vi "6.1 Cluster to CSM API String.vi"() -> ()   [LabVIEW 2017]
doc: "### 6.1 Cluster to CSM API String.vi\n\n#### Overview\n\nDemonstrates API String expression for a cluster.\n\n#### Introduction\n\nA cluster is a complex type composed of other data types. This example shows API String expression for clusters. In an API String, a cluster can be expressed in the following two ways:\n\n1. **Tag:Value Mode** In Tag:Value mode, the input string consists of multiple tag-value pairs. A colon (`:`) separates the tag and data, and a semicolon (`;`) separates different elements. Curly braces (`{` and `}`) are used as boundary symbols. For non-complex mixed data types, curly braces can be omitted.\n2. **No-Tag Mode** Clusters also support inputting only data strings, with values separated by semicolons.\n\n#### Steps\n\n- step1: Tag:Value Mode.\n- step2: No-Tag Mode."
uses:
  601d0760-d4b8-4795-a453-687868710894.vi
  39620bd7-9c21-4071-a996-c10094c7c5f6.vi
  6aef6293-1b46-43cc-a090-3bd41170cef4.vi
  c2ea3052-9718-4095-9bf2-a156dcd4a46a.vi
  addons/API-String-Arugments-Support/_Support/Data To API String Arguments.vi
  addons/API-String-Arugments-Support/_Support/Convert API String Arguments to Data(variant).vi
panel:
  out "output cluster":T1={"Data 8"={"Name"="abc", "Child"={"Name"="xxx"}, "Bool"=TRUE}, "Reference cluster in Flatten"={"Name"="abc", "Child"={"Name"="ddd"}, "Bool"=FALSE}, "Flattened String"="{Child.Name:xxx;Bool:TRUE}", "Reference cluster in Retrieve"={"Name"="abc", "Child"={"Name"="ddd"}, "Bool"=FALSE}, "Retrieved Data"={"Name"="abc", "Child"={"Name"="xxx"}, "Bool"=TRUE}}
  out "Flatten Without Reference Cluster":T2={"Original Data"={"Name"="abc", "Child"={"Name"="ddd"}, "Bool"=FALSE}, "Default Reference in Flatten"=variant, "Flattened String"="{Name:abc;Child.Name:ddd;Bool:FALSE}", "Reference cluster in Retrieve"={"Name"="abc", "Child"={"Name"="ddd"}, "Bool"=FALSE}, "Retrieved Data"={"Name"="abc", "Child"={"Name"="ddd"}, "Bool"=FALSE}}
  # "#CSM-Example Overview\n\nDemonstrates API String expression for a cluster."
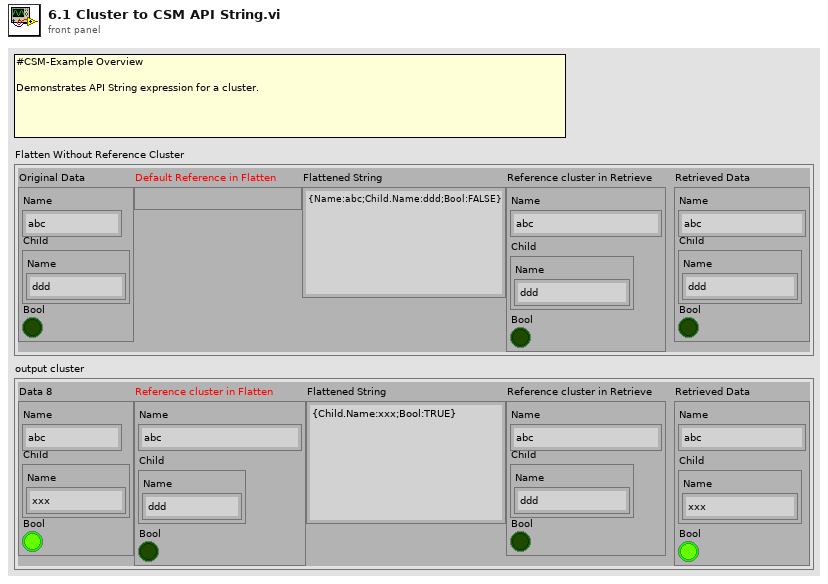
[diagram p1: front panel]
types:
  T1 = cluster{"Data 8":cluster{"Name":string, "Child":cluster{"Name":string}, "Bool":bool}, "Reference cluster in Flatten":cluster{"Name":string, "Child":cluster{"Name":string}, "Bool":bool}, "Flattened String":string, "Reference cluster in Retrieve":cluster{"Name":string, "Child":cluster{"Name":string}, "Bool":bool}, "Retrieved Data":cluster{"Name":string, "Child":cluster{"Name":string}, "Bool":bool}}
  T2 = cluster{"Original Data":cluster{"Name":string, "Child":cluster{"Name":string}, "Bool":bool}, "Default Reference in Flatten":variant, "Flattened String":string, "Reference cluster in Retrieve":cluster{"Name":string, "Child":cluster{"Name":string}, "Bool":bool}, "Retrieved Data":cluster{"Name":string, "Child":cluster{"Name":string}, "Bool":bool}}
  T3 = cluster{"Name":string, "Child":cluster{"Name":string}, "Bool":bool}
  T4 = cluster{"Data 8":cluster{"Name":string, "Child":cluster{"Name":string}, "Bool":bool}, "reference cluster data":variant, "API String":string, "Reference cluster data":cluster{"Name":string, "Child":cluster{"Name":string}, "Bool":bool}, "Data":cluster{"Name":string, "Child":cluster{"Name":string}, "Bool":bool}}
  T5 = cluster{"Data 8":cluster{"Name":string, "Child":cluster{"Name":string}, "Bool":bool}, "Reference cluster data":cluster{"Name":string, "Child":cluster{"Name":string}, "Bool":bool}, "API String":string, "Reference cluster data":cluster{"Name":string, "Child":cluster{"Name":string}, "Bool":bool}, "Data":cluster{"Name":string, "Child":cluster{"Name":string}, "Bool":bool}}
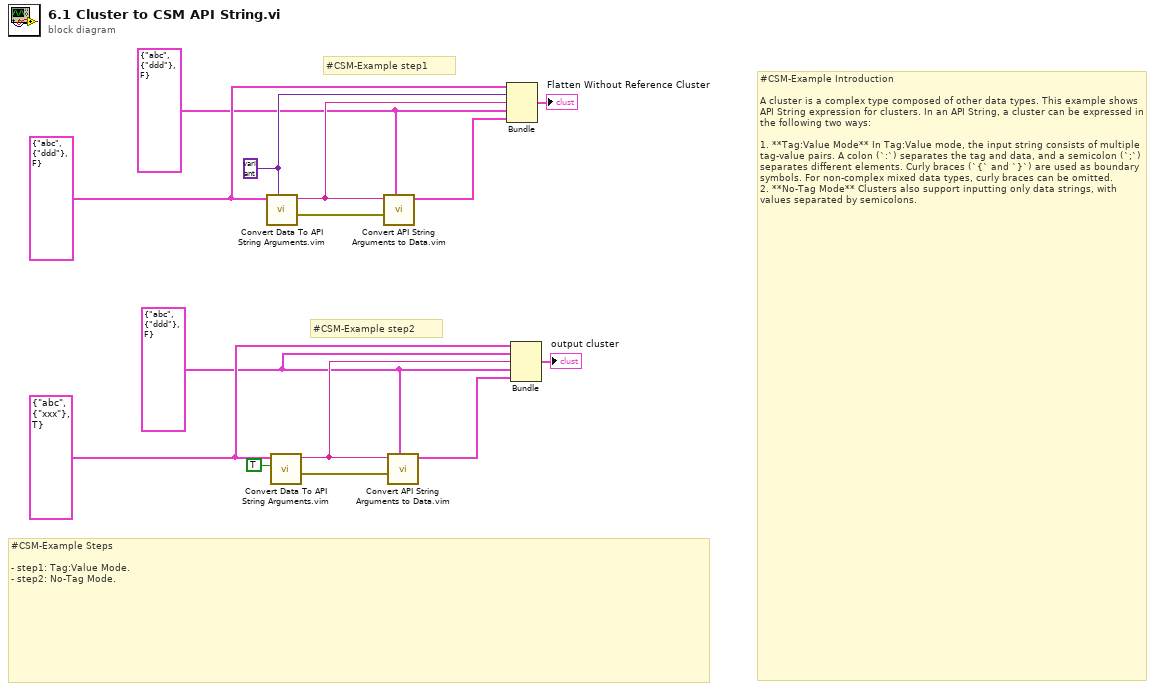
[diagram p0: block diagram]
diagram:
  w3 = T3 {"Name"="abc", "Child"={"Name"="ddd"}, "Bool"=FALSE} ("Reference cluster data")
  w5 = T3 {"Name"="abc", "Child"={"Name"="xxx"}, "Bool"=TRUE} ("Data 8")
  w10 = T3 {"Name"="abc", "Child"={"Name"="ddd"}, "Bool"=FALSE} ("Reference cluster data")
  w12 = variant ("reference cluster data")
  w13 = T3 {"Name"="abc", "Child"={"Name"="ddd"}, "Bool"=FALSE} ("Data 8")
  # "#CSM-Example step2"
  # "#CSM-Example step1"
  # "#CSM-Example Steps\n\n- step1: Tag:Value Mode.\n- step2: No-Tag Mode."
  # "#CSM-Example Introduction\n\nA cluster is a complex type composed of other data types. This example shows API String expression for clusters. In an API String, a cluster can be expressed in the following two ways:\n\n1. **Tag:Value Mode** In Tag:Value mode, the input string consists of multiple tag-value pairs. A colon (`:`) separates the tag and data, and a semicolon (`;`) separates different elements. Curly braces (`{` and `}`) are used as boundary symbols. For non-complex mixed data types, curly braces can be omitted.\n2. **No-Tag Mode** Clusters also support inputting only data strings, with values separated by semicolons."
  n1 = call "Convert Data To API String Arguments.vim"("Reference Cluster Data"=w12, "Data"=w13) -> ("error out"=w14:errorcluster, "API String"=w11:string)  [unwired: 6 in]
  n2 = call "Convert Data To API String Arguments.vim"("No Tag Mode? (F)"=TRUE ("No Tag Mode(F)"), "Data"=w5) -> ("error out"=w4:errorcluster, "API String"=w6:string)  [unwired: 6 in]
  n3 = call "Convert API String Arguments to Data.vim"("Reference Type"=w10, "error in (no error)"=w14, "API String"=w11) -> ("Data"=w9:T3)  [unwired: 5 in, 1 out]
  n4 = call "Convert API String Arguments to Data.vim"("Reference Type"=w3, "error in (no error)"=w4, "API String"=w6) -> ("Data"=w7:T3)  [unwired: 5 in, 1 out]
  n5 = Bundle("Data 8"=w13, "reference cluster data"=w12, "API String"=w11, "Reference cluster data"=w10, "Data"=w9) -> (→"Flatten Without Reference Cluster":T4)  [unwired: 1 in]
  n6 = Bundle("Data 8"=w5, "Reference cluster data"=w3, "API String"=w6, "Reference cluster data"=w3, "Data"=w7) -> (→"output cluster":T5)  [unwired: 1 in]
